vi "ZDataVIS_ScaleSelect.vi"(4 "Manual CTLs":T1={"X Low"=-0.1, "X High"=0.1, "X Step Size"=4e-05} {"X Step Size" format="%#_6p"; "X High" format="%#_6p"; "X Low" format="%#_6p"}, 6 "Auto CTLs":cluster{"METHOD":bool, "Steps":dbl}, 8 "error in (no error)":errorcluster, 10 "X Scale Selection 2":enum32{"Manual", "Auto"}(tab), 11 "Intensity Info IN":cluster{dbl[], dbl[]}[](array[cluster])) -> (0 "error out":errorcluster, 2 "X Step Info":cluster{"X Low":dbl, "X High":dbl, "X Step":dbl}={"X Low"=-0.1, "X High"=0.1, "X Step"=4e-05} {"X Step" format="%#_6p"; "X High" format="%#_6p"; "X Low" format="%#_6p"}, 3 "Intensity InfoOUT":cluster{dbl[], dbl[]}[](array[cluster]))   [LabVIEW 2016]
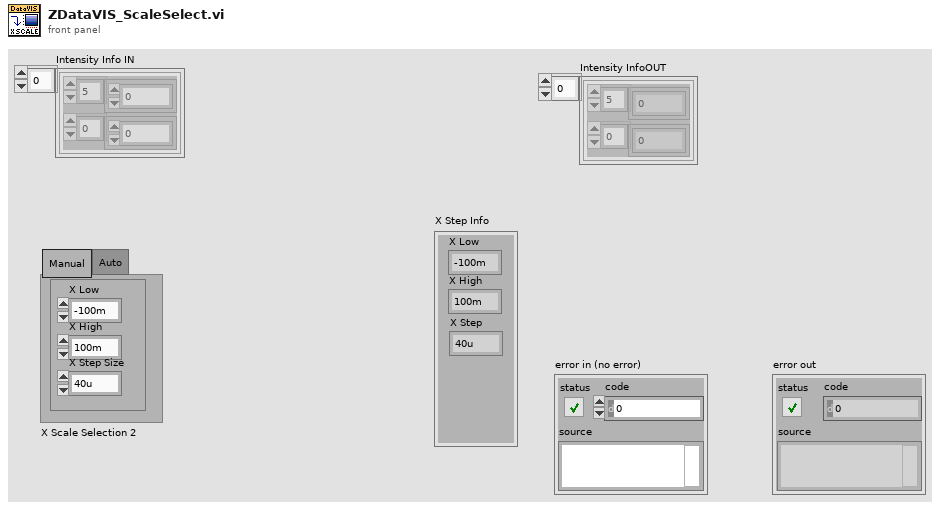
[diagram p1: front panel]
types:
  T1 = cluster{"X Low":dbl, "X High":dbl, "X Step Size":dbl}
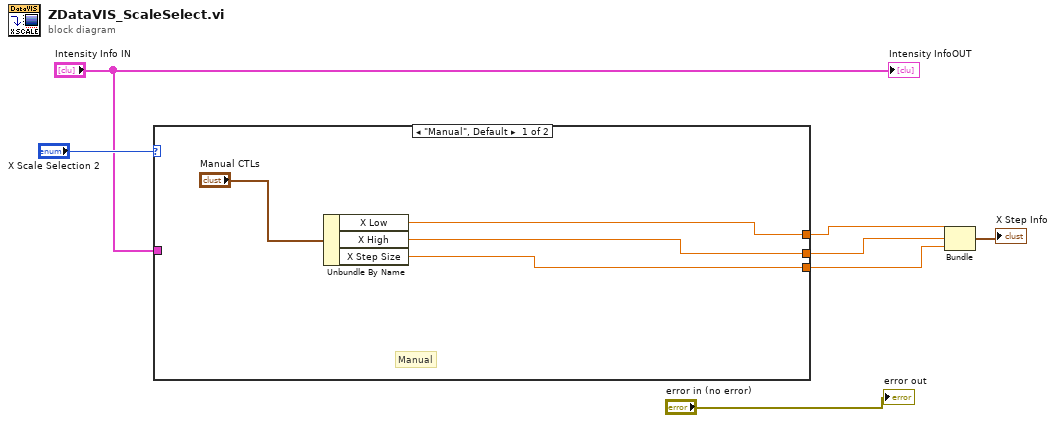
[diagram p0: block diagram]
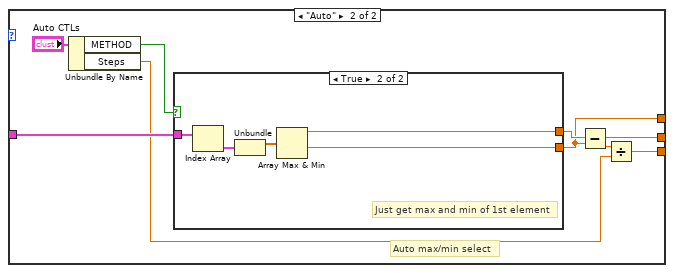
[diagram p2: hidden frame]
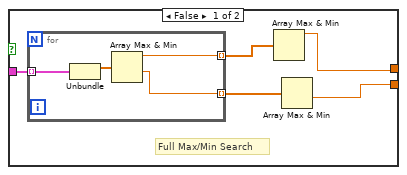
[diagram p3: hidden frame]
diagram:
  n1 = case shown="\"Manual\", Default" "X Scale Selection 2" {
    tunnel: [w8 w15] -> w5
    tunnel: [w10 w17] -> w3
    tunnel: [w9 w18] -> w4
    tunnel: "Intensity Info IN" -> [_ w19]
    frame "Manual", Default {
      # "Manual"
      n2 = Unbundle By Name("Manual CTLs") -> ("X Low"=w10:dbl, "X High"=w9:dbl, "X Step Size"=w8:dbl)
    }
    frame "Auto" {
      # "Auto max/min select"
      n3 = Unbundle By Name("Auto CTLs") -> ("METHOD"=w13:bool, "Steps"=w12:dbl)
      n4 = case shown="True" w13 {
        tunnel: [w20 w30] -> w17
        tunnel: [w21 w29] -> w18
        tunnel: w19 -> [w24 w33]
        frame False {
          # "Full Max/Min Search"
          n5 = for {
            tunnel: w24 -> [w27] mode=indexing
            tunnel: [w26] -> w23 mode=indexing
            tunnel: [w25] -> w22 mode=indexing
            n6 = Unbundle(w27) -> (w28:dbl[])  [unwired: 1 out]
            n7 = Array Max & Min(array=w28) -> (max value=w26:dbl, min value=w25:dbl)  [unwired: 2 out]
          }
          n8 = Array Max & Min(array=w23) -> (max value=w21:dbl)  [unwired: 3 out]
          n9 = Array Max & Min(array=w22) -> (min value=w20:dbl)  [unwired: 3 out]
        }
        frame True {
          # "Just get max and min of 1st element"
          n10 = Index Array(array=w33) -> (element=w32:cluster{dbl[], dbl[]})  [unwired: 1 in]
          n11 = Unbundle(w32) -> (w31:dbl[])  [unwired: 1 out]
          n12 = Array Max & Min(array=w31) -> (max value=w29:dbl, min value=w30:dbl)  [unwired: 2 out]
        }
      }
      n13 = Subtract(x=w18, y=w17) -> (x-y=w16:dbl)
      n14 = Divide(x=w16, y=w12) -> (x/y=w15:dbl)
    }
  }
  n15 = Bundle("X Low"=w3, "X High"=w4, "X Step Size"=w5) -> (→"X Step Info":T1)  [unwired: 1 in]
  "error out" <- "error in (no error)"
  "Intensity InfoOUT" <- "Intensity Info IN"
